vi "Save_LDA_Channel_Setup.vi"() -> (0 "Setup file string":string)   [LabVIEW 2022 SP3]
uses:
  Globals/LDA_global.vi
  Globals/Meas_global.vi
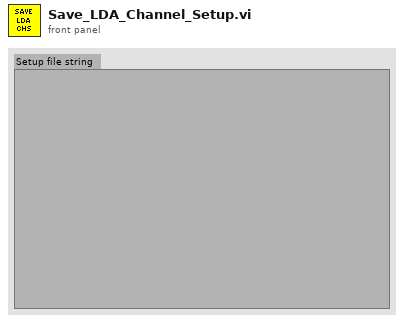
[diagram p1: front panel]
types:
  T1 = typedef "LDA_Channel.ctl" = cluster{"Wavelength (nm)":dbl, "Vel Comp":string, "Max Velocity":dbl, "Min Velocity":dbl, "Max Record length":u16, "Signal gain (dB)":i16, "High voltage":i16, "Optics Conversion Factor":dbl, "Min Record length":u16, "Multiply Velocity by -1":bool, "Signal to Noise Ratio":string, "Validation Ratio":string, "Probe":string, "Laser":string, "BSA":string, "Lense":string, "Beam Separation (mm)":dbl, "Focal Length (mm)":dbl, "COLOUR":u32, "BSA IP":string, "Velocity Range (m/s)":dbl, "Centre Velocity (m/s)":dbl, "Unshifted mW":dbl, "Shifted mW":dbl, "Bandwidth Hz":dbl, "Req Sampling Rate Hz":dbl, "Ch":i32, "CenterFreq Hz":dbl, "Laser IP":string, "Sync Delay (s)":dbl}
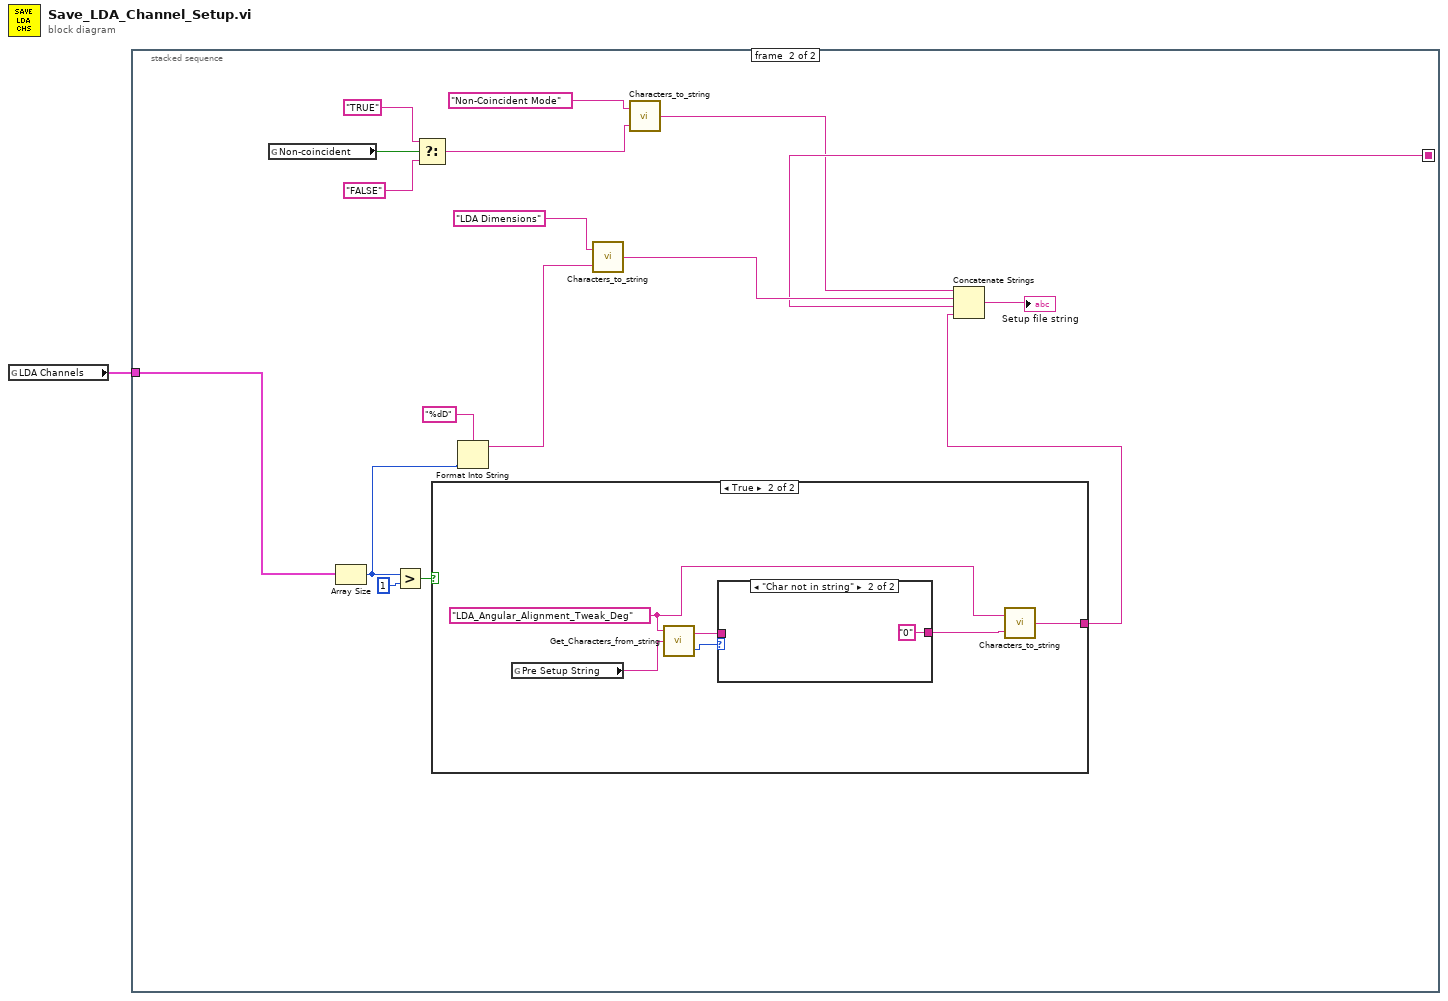
[diagram p0: block diagram]
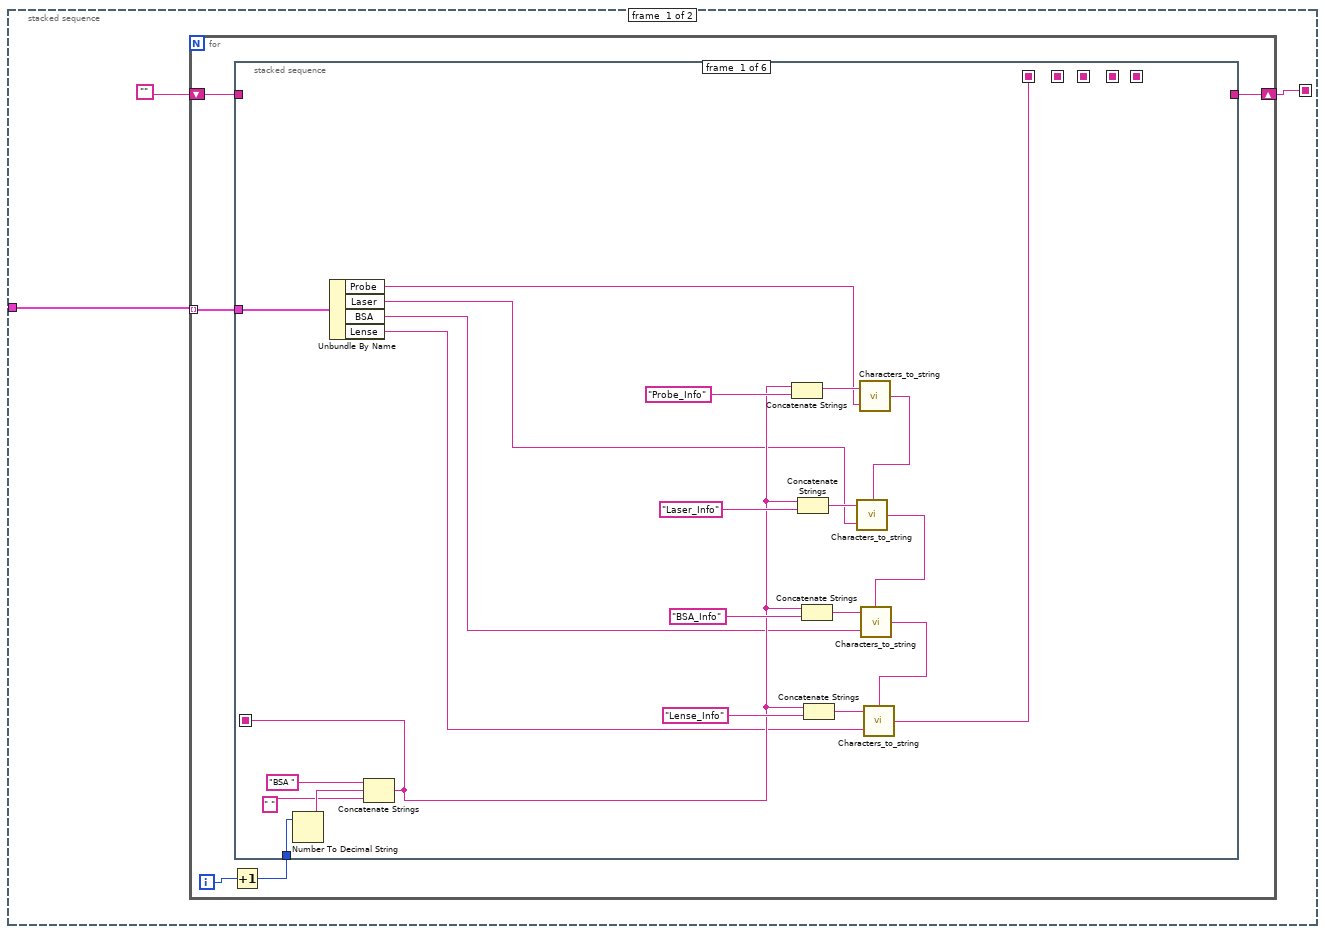
[diagram p2: hidden frame]
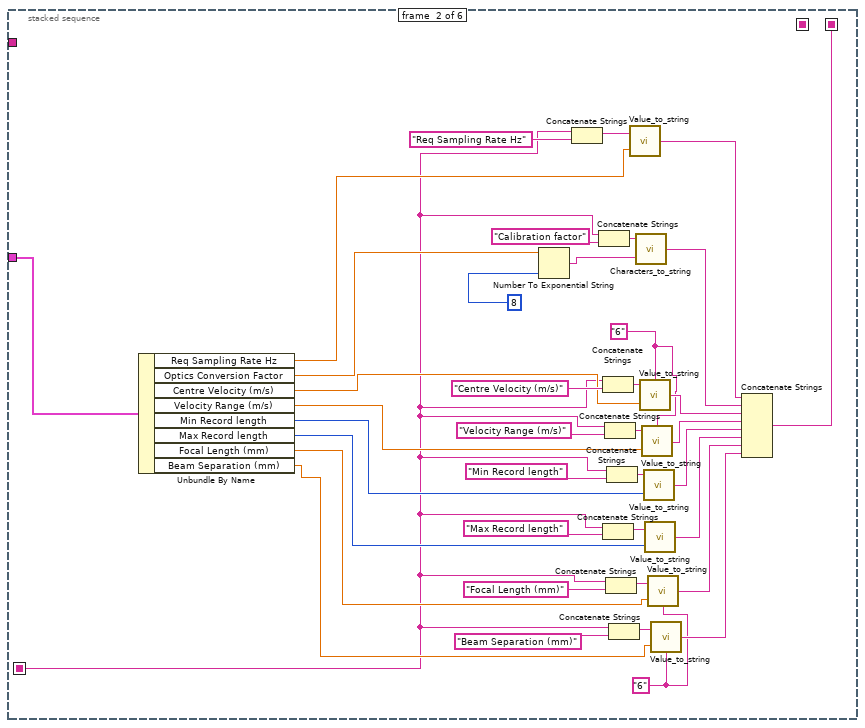
[diagram p3: hidden frame]
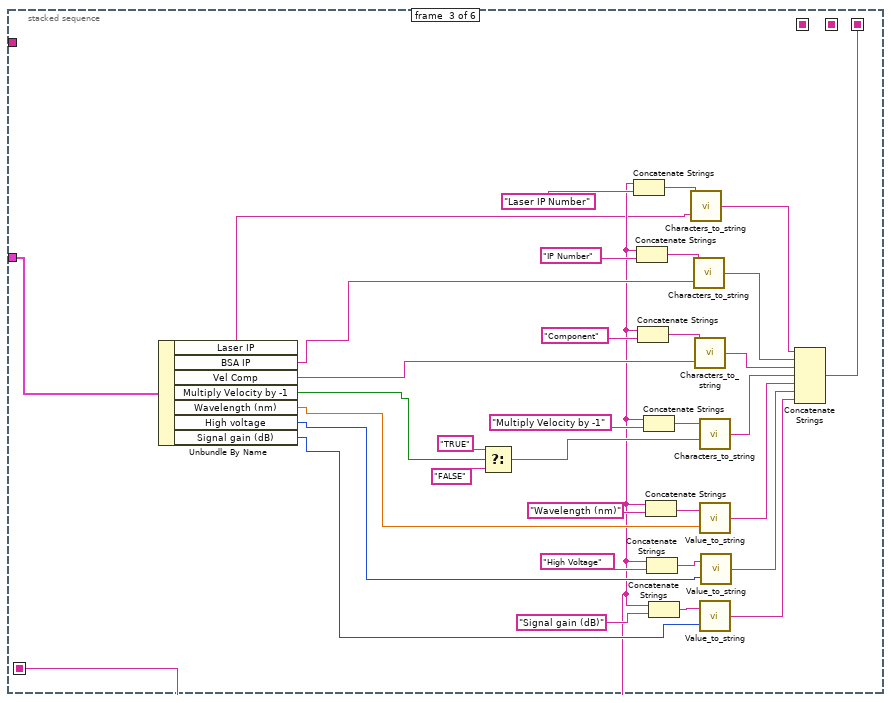
[diagram p4: hidden frame]
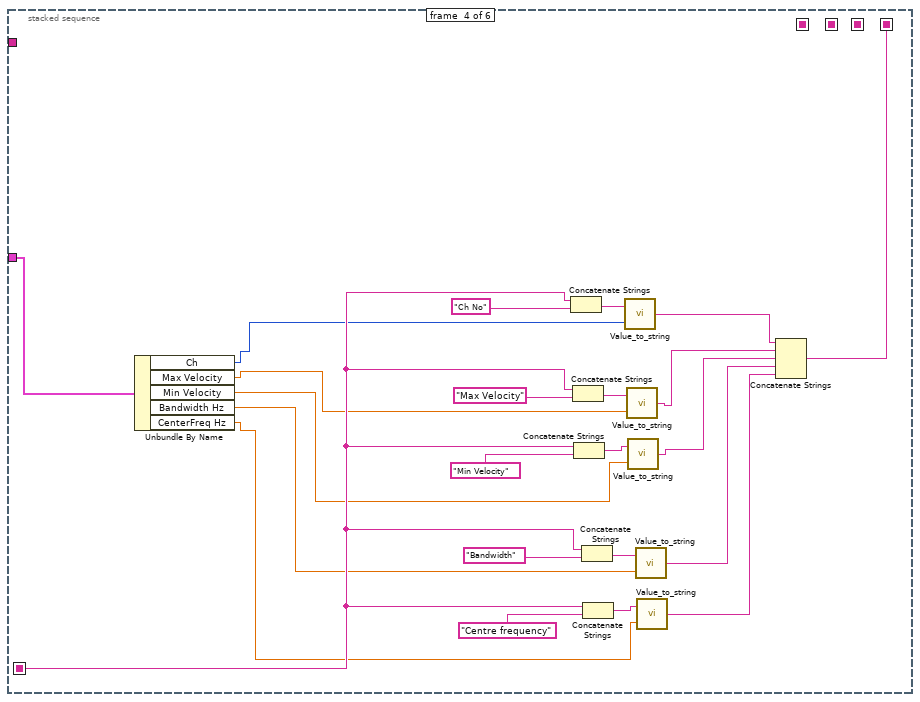
[diagram p5: hidden frame]
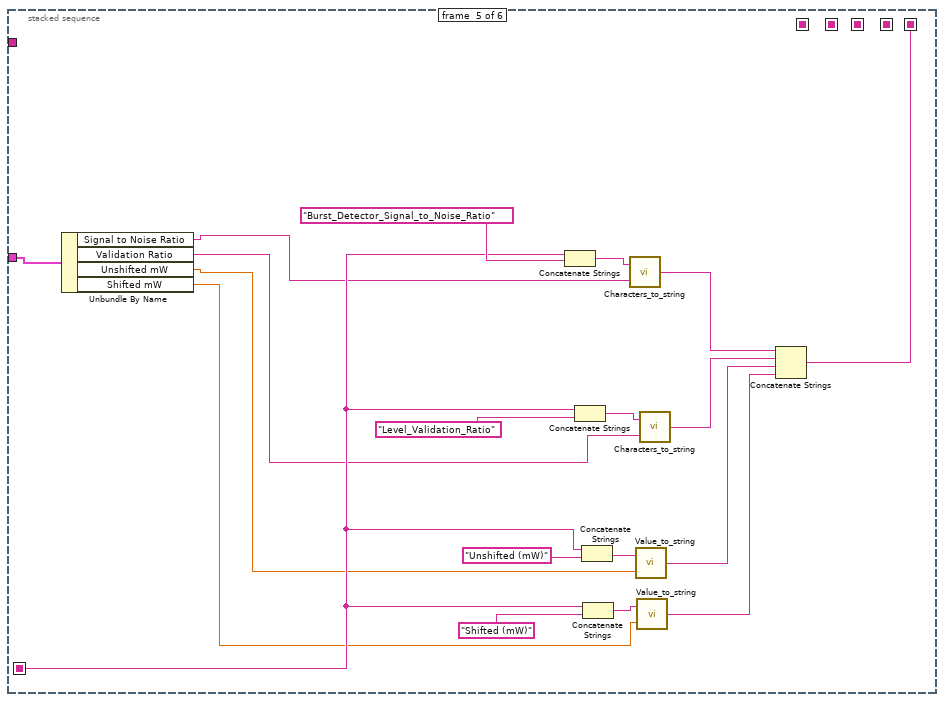
[diagram p6: hidden frame]
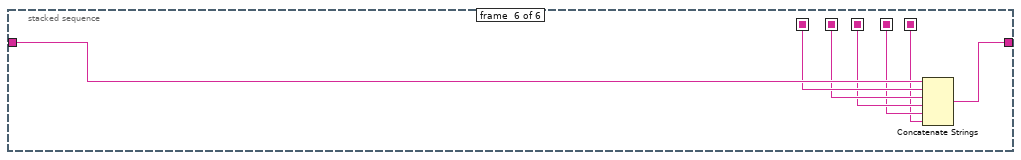
[diagram p7: hidden frame]
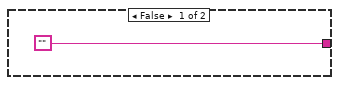
[diagram p8: hidden frame]
diagram:
  n1 = global read "LDA_global.vi" "LDA Channels"() -> (w1:T1[])
  n2 = stacked-sequence {
    seq-local: [w2 _] -> [_ w162]
    tunnel: w1 -> [w3 w164]
    frame #0 {
      n3 = for {
        shift-right: [w6] -> w2
        shift-left: "" -> [w7]
        tunnel: w3 -> [w5] mode=indexing
        i -> [w9]
        n4 = Increment(x=w9) -> (x+1=w8:i32)
        n5 = stacked-sequence {
          seq-local: [w19 _ _ _ _ _] -> [_ w34 w72 w111 w134 _]
          seq-local: [w10 _ _ _ _ _] -> [_ _ _ _ _ w152]
          seq-local: [_ w45 _ _ _ _] -> [_ _ _ _ _ w151]
          seq-local: [_ _ w86 _ _ _] -> [_ _ _ _ _ w149]
          seq-local: [_ _ _ w127 _ _] -> [_ _ _ _ _ w148]
          seq-local: [_ _ _ _ w133 _] -> [_ _ _ _ _ w147]
          tunnel: w8 -> [w28 _ _ _ _ _]
          tunnel: w7 -> [_ _ _ _ _ w153]
          tunnel: [_ _ _ _ _ w150] -> w6
          tunnel: w5 -> [w18 w44 w82 w110 w132 _]
          frame #0 {
            n6 = Number To Decimal String(number=w28) -> (decimal integer string=w31:string)  [unwired: 1 out]
            n7 = Unbundle By Name(w18) -> ("Probe"=w17:string, "Laser"=w16:string, "BSA"=w14:string, "Lense"=w15:string)
            n8 = Concatenate Strings("BSA ", w31, " ") -> (w19:string)
            n9 = Concatenate Strings(w19, "Probe_Info" ("Pre Setup String")) -> (w25:string)
            n10 = Concatenate Strings(w19, "Laser_Info" ("string")) -> (w26:string)
            n11 = Concatenate Strings(w19, "BSA_Info" ("string")) -> (w23:string)
            n12 = Concatenate Strings(w19, "Lense_Info" ("string")) -> (w20:string)
            n13 = call "Characters_to_string.vi"("Characters to write"=w17, "Label for characters"=w25) -> ("Output string"=w13:string)  [unwired: 1 in]
            n14 = call "Characters_to_string.vi"("stringIn"=w13, "Characters to write"=w16, "Label for characters"=w26) -> ("Output string"=w12:string)
            n15 = call "Characters_to_string.vi"("stringIn"=w12, "Characters to write"=w14, "Label for characters"=w23) -> ("Output string"=w11:string)
            n16 = call "Characters_to_string.vi"("stringIn"=w11, "Characters to write"=w15, "Label for characters"=w20) -> ("Output string"=w10:string)
          }
          frame #1 {
            w46 = "6" ("precision")
            w47 = "6" ("precision")
            n17 = Unbundle By Name(w44) -> ("Req Sampling Rate Hz"=w36:dbl, "Optics Conversion Factor"=w43:dbl, "Centre Velocity (m/s)"=w42:dbl, "Velocity Range (m/s)"=w41:dbl, "Min Record length"=w40:u16, "Max Record length"=w39:u16, "Focal Length (mm)"=w38:dbl, "Beam Separation (mm)"=w37:dbl)
            n18 = Number To Exponential String(number=w43, precision (6)=i16 8) -> (E-format string=w64:string)  [unwired: 2 out]
            n19 = Concatenate Strings(w34, "Req Sampling Rate Hz") -> (w33:string)
            n20 = Concatenate Strings(w34, "Calibration factor") -> (w48:string)
            n21 = Concatenate Strings(w34, "Centre Velocity (m/s)") -> (w49:string)
            n22 = Concatenate Strings(w34, "Max Record length") -> (w61:string)
            n23 = Concatenate Strings(w34, "Velocity Range (m/s)") -> (w50:string)
            n24 = Concatenate Strings(w34, "Focal Length (mm)" ("Label for characters")) -> (w65:string)
            n25 = Concatenate Strings(w34, "Min Record length") -> (w51:string)
            n26 = Concatenate Strings(w34, "Beam Separation (mm)" ("Label for characters")) -> (w66:string)
            n27 = call "Value_to_string.vi"("Value"=w36, "Label for value"=w33) -> ("Output string"=w32:string)  [unwired: 1 in]
            n28 = call "Characters_to_string.vi"("Characters to write"=w64, "Label for characters"=w48) -> ("Output string"=w52:string)  [unwired: 1 in]
            n29 = call "Value_to_string.vi"("precision"=w46, "Value"=w42, "Label for value"=w49) -> ("Output string"=w53:string)
            n30 = call "Value_to_string.vi"("precision"=w46, "Value"=w41, "Label for value"=w50) -> ("Output string"=w54:string)
            n31 = call "Value_to_string.vi"("Value"=w40, "Label for value"=w51) -> ("Output string"=w59:string)  [unwired: 1 in]
            n32 = call "Value_to_string.vi"("Value"=w39, "Label for value"=w61) -> ("Output string"=w62:string)  [unwired: 1 in]
            n33 = call "Value_to_string.vi"("precision"=w47, "Value"=w38, "Label for value"=w65) -> ("Output string"=w69:string)
            n34 = call "Value_to_string.vi"("precision"=w47, "Value"=w37, "Label for value"=w66) -> ("Output string"=w70:string)
            n35 = Concatenate Strings(w32, w52, w53, w54, w59, w62, w69, w70) -> (w45:string)
          }
          frame #2 {
            n36 = Unbundle By Name(w82) -> ("Laser IP"=w71:string, "BSA IP"=w81:string, "Vel Comp"=w80:string, "Multiply Velocity by -1"=w79:bool, "Wavelength (nm)"=w78:dbl, "High voltage"=w77:i16, "Signal gain (dB)"=w76:i16)
            n37 = Select(t="TRUE" ("y"), s=w79, f="FALSE" ("y")) -> (s? t:f=w94:string)
            n38 = Concatenate Strings(w72, "Laser IP Number") -> (w74:string)
            n39 = Concatenate Strings(w72, "IP Number") -> (w85:string)
            n40 = Concatenate Strings(w72, "Component") -> (w87:string)
            n41 = Concatenate Strings(w72, "Multiply Velocity by -1") -> (w91:string)
            n42 = Concatenate Strings(w72, "Wavelength (nm)") -> (w96:string)
            n43 = Concatenate Strings(w72, "High Voltage") -> (w97:string)
            n44 = Concatenate Strings(w72, "Signal gain (dB)") -> (w98:string)
            n45 = call "Characters_to_string.vi"("Characters to write"=w71, "Label for characters"=w74) -> ("Output string"=w73:string)  [unwired: 1 in]
            n46 = call "Characters_to_string.vi"("Characters to write"=w81, "Label for characters"=w85) -> ("Output string"=w83:string)  [unwired: 1 in]
            n47 = call "Characters_to_string.vi"("Characters to write"=w80, "Label for characters"=w87) -> ("Output string"=w88:string)  [unwired: 1 in]
            n48 = call "Characters_to_string.vi"("Characters to write"=w94, "Label for characters"=w91) -> ("Output string"=w95:string)  [unwired: 1 in]
            n49 = call "Value_to_string.vi"("Value"=w78, "Label for value"=w96) -> ("Output string"=w103:string)  [unwired: 1 in]
            n50 = call "Value_to_string.vi"("Value"=w76, "Label for value"=w98) -> ("Output string"=w101:string)  [unwired: 1 in]
            n51 = call "Value_to_string.vi"("Value"=w77, "Label for value"=w97) -> ("Output string"=w102:string)  [unwired: 1 in]
            n52 = Concatenate Strings(w73, w83, w88, w95, w103, w102, w101) -> (w86:string)
          }
          frame #3 {
            n53 = Unbundle By Name(w110) -> ("Ch"=w109:i32, "Max Velocity"=w108:dbl, "Min Velocity"=w107:dbl, "Bandwidth Hz"=w106:dbl, "CenterFreq Hz"=w105:dbl)
            n54 = Concatenate Strings(w111, "Ch No") -> (w113:string)
            n55 = Concatenate Strings(w111, "Max Velocity") -> (w120:string)
            n56 = Concatenate Strings(w111, "Min Velocity") -> (w119:string)
            n57 = Concatenate Strings(w111, "Bandwidth") -> (w123:string)
            n58 = Concatenate Strings(w111, "Centre frequency") -> (w124:string)
            n59 = call "Value_to_string.vi"("Value"=w109, "Label for value"=w113) -> ("Output string"=w112:string)  [unwired: 1 in]
            n60 = call "Value_to_string.vi"("Value"=w108, "Label for value"=w120) -> ("Output string"=w115:string)  [unwired: 1 in]
            n61 = call "Value_to_string.vi"("Value"=w107, "Label for value"=w119) -> ("Output string"=w116:string)  [unwired: 1 in]
            n62 = call "Value_to_string.vi"("Value"=w106, "Label for value"=w123) -> ("Output string"=w122:string)  [unwired: 1 in]
            n63 = call "Value_to_string.vi"("Value"=w105, "Label for value"=w124) -> ("Output string"=w121:string)  [unwired: 1 in]
            n64 = Concatenate Strings(w112, w115, w116, w122, w121) -> (w127:string)
          }
          frame #4 {
            n65 = Unbundle By Name(w132) -> ("Signal to Noise Ratio"=w131:string, "Validation Ratio"=w130:string, "Unshifted mW"=w129:dbl, "Shifted mW"=w128:dbl)
            n66 = Concatenate Strings(w134, "Burst_Detector_Signal_to_Noise_Ratio" ("Pre Setup String")) -> (w142:string)
            n67 = Concatenate Strings(w134, "Level_Validation_Ratio" ("Pre Setup String")) -> (w143:string)
            n68 = Concatenate Strings(w134, "Unshifted (mW)") -> (w137:string)
            n69 = Concatenate Strings(w134, "Shifted (mW)") -> (w138:string)
            n70 = call "Characters_to_string.vi"("Characters to write"=w131, "Label for characters"=w142) -> ("Output string"=w146:string)  [unwired: 1 in]
            n71 = call "Value_to_string.vi"("Value"=w129, "Label for value"=w137) -> ("Output string"=w136:string)  [unwired: 1 in]
            n72 = call "Value_to_string.vi"("Value"=w128, "Label for value"=w138) -> ("Output string"=w135:string)  [unwired: 1 in]
            n73 = call "Characters_to_string.vi"("Characters to write"=w130, "Label for characters"=w143) -> ("Output string"=w145:string)  [unwired: 1 in]
            n74 = Concatenate Strings(w146, w145, w136, w135) -> (w133:string)
          }
          frame #5 {
            n75 = Concatenate Strings(w153, w152, w151, w149, w148, w147) -> (w150:string)
          }
        }
      }
    }
    frame #1 {
      n76 = global read "LDA_global.vi" "Non-coincident"() -> (w157:bool)
      n77 = Array Size(array=w164) -> (size(s)=w167:i32)
      n78 = Greater?(x=w167, y=1) -> (0:w166:bool)
      n79 = Select(t="TRUE", s=w157, f="FALSE") -> (s? t:f=w154:string)
      n80 = case shown="True" w166 {
        tunnel: ["" w175] -> w161
        frame False {
        }
        frame True {
          w174 = "LDA_Angular_Alignment_Tweak_Deg"
          n81 = global read "Meas_global.vi" "Pre Setup String"() -> (w176:string)
          n82 = call "Get_Characters_from_string.vi"("Input string"=w176, "Variable name"=w174) -> ("Status"=w177:enum16{"Char in string", "Char not in string"}, "Value"=w172:string)  [unwired: 1 in]
          n83 = case shown="\"Char not in string\"" w177 {
            tunnel: [w178 "0" ("Value")] -> w173
            tunnel: w172 -> [w178 _]
            frame "Char in string" {
            }
            frame "Char not in string" {
            }
          }
          n84 = call "Characters_to_string.vi"("Characters to write"=w173, "Label for characters"=w174) -> ("Output string"=w175:string)  [unwired: 1 in]
        }
      }
      n85 = Format Into String(format string="%dD", w167) -> (resulting string=w169:string)  [unwired: 2 in, 1 out]
      n86 = call "Characters_to_string.vi"("Characters to write"=w169, "Label for characters"="LDA Dimensions") -> ("Output string"=w163:string)  [unwired: 1 in]
      n87 = call "Characters_to_string.vi"("Characters to write"=w154, "Label for characters"="Non-Coincident Mode" ("Pre Setup String")) -> ("Output string"=w158:string)  [unwired: 1 in]
      n88 = Concatenate Strings(w158, w163, w162, w161) -> (→"Setup file string":string)
    }
  }
